vi "Write Current Waveform to Log Instances.vi"(6 "Current Wfm":T1, 8 "error in (no error)":errorcluster, 9 "Data in":dbl[](array[numeric]), 10 "Wfm Index":i32, 11 "Waveform Log in":refnum<class "Waveform Log.lvclass">) -> (0 "error out":errorcluster, 1 "Data out":dbl[](array[numeric]), 3 "Waveform Log out":refnum<class "Waveform Log.lvclass">)   [LabVIEW 2015, in "Waveform Data Logger Engine.lvlib" / "Waveform Log.lvclass"]
uses:
  Waveform Log.lvclass
  Waveform Receive/Wfm Info.ctl
  Waveform Log.lvclass/Waveform Log.ctl
  Logs/Segmented Logs/Segmented Log/Segmented Log.lvclass/Segmented Log.ctl
  Shared/Classes/Log File Specifications/Log File Specification/Log File Specification.lvclass/Log File Specification.ctl
  Shared/Classes/Log File Specifications/Waveform TDMS Log File Specification/Waveform TDMS Log File Specification.lvclass/Waveform TDMS Log File Specification.ctl
  Logs/Log Files/Log File/Log File.lvclass/Log File.ctl
  Logs/Log Files/TDMS Log File/TDMS Log File.lvclass/TDMS Log File.ctl
  Logs/Log Files/Text Log File/Text Log File.lvclass/Text Log File.ctl
  Logs/Segmented Logs/Footprint Segmented Log/Footprint Segmented Log.lvclass/Footprint Segmented Log.ctl
  Logs/Segmented Logs/Time Segmented Log/Time Segmented Log.lvclass/Time Segmented Log.ctl
  Logs/Segmented Logs/Segmented Log/Write Waveform to Log File Instance.vi
  Shared/Classes/Log File Specifications/Log File Specification/Get Log Specification Type.vi
  Shared/Classes/Log File Specifications/Waveform TDMS Log File Specification/Get Current Group.vi
  Logs/Log Files/Log File/Get Log File Type.vi
  Logs/Log Files/Log File/Write Channel to Log File.vi
  Logs/Log Files/TDMS Log File/Set TDMS Channel Property.vi
  Logs/Log Files/TDMS Log File/Copy Channel Properties.vi
  Logs/Segmented Logs/Segmented Log/Check Close File.vi
  Logs/Segmented Logs/Segmented Log/Check Open File.vi
  Logs/Log Files/TDMS Log File/Write Channel to TDMS Log File.vi
  Logs/Log Files/Text Log File/Write Channel to Text Log File.vi
  Logs/Segmented Logs/Segmented Log/Close Log File Instance.vi
  Logs/Segmented Logs/Segmented Log/Segment Log File.vi
  Logs/Segmented Logs/Segmented Log/Open Log File Instance.vi
  Logs/Log Files/Log File/Close Log File.vi
  Logs/Segmented Logs/Segmented Log/Make File Read-Only.vi
  Logs/Segmented Logs/Segmented Log/On Segmented Log Complete.vi
  Logs/Segmented Logs/Segmented Log/On File Close.vi
  Logs/Segmented Logs/Footprint Segmented Log/Segment Log File (Footprint).vi
  Logs/Segmented Logs/Time Segmented Log/Segment Log File (Time).vi
  Shared/Classes/Log File Specifications/Log File Specification/Open Log File.vi
  Shared/Classes/Log File Specifications/Log File Specification/Set Path Tag.vi
  Logs/Segmented Logs/Segmented Log/On File Open.vi
  Shared/Classes/Log File Specifications/Log File Specification/Set Filename Offset.vi
  Logs/Log Files/TDMS Log File/Close TDMS Log File.vi
  Logs/Log Files/Text Log File/Close Text Log File.vi
  Logs/Segmented Logs/Segmented Log/Get Current Log File Instance.vi
  Logs/Log Files/Log File/Get File Size.vi
  Logs/Log Files/Log File/Get Start Time.vi
  Shared/Classes/Log File Specifications/Log File Specification/Build File Path.vi
  Shared/Classes/Log File Specifications/Log File Specification/Resolve File Conflicts.vi
  <vilib>/Utility/error.llb/Error Cluster From Error Code.vi
  Shared/Classes/Log File Specifications/Log File Specification/Initialize Log File.vi
  <vilib>/Utility/libraryn.llb/Create Directory Recursive.vi
  <vilib>/Utility/libraryn.llb/Check if File or Folder Exists.vi
  <vilib>/Utility/libraryn.llb/Get File Extension.vi
  Logs/Log Files/Text Log File/Text Log File.lvclass
  Logs/Log Files/TDMS Log File/TDMS Log File.lvclass
  Logs/Log Files/Log File/Log File.lvclass
  Logs/Segmented Logs/Time Segmented Log/Time Segmented Log.lvclass
  Logs/Segmented Logs/Footprint Segmented Log/Footprint Segmented Log.lvclass
  Shared/Classes/Log File Specifications/Waveform TDMS Log File Specification/Waveform TDMS Log File Specification.lvclass
  Waveform Receive/Waveform Receive.lvclass
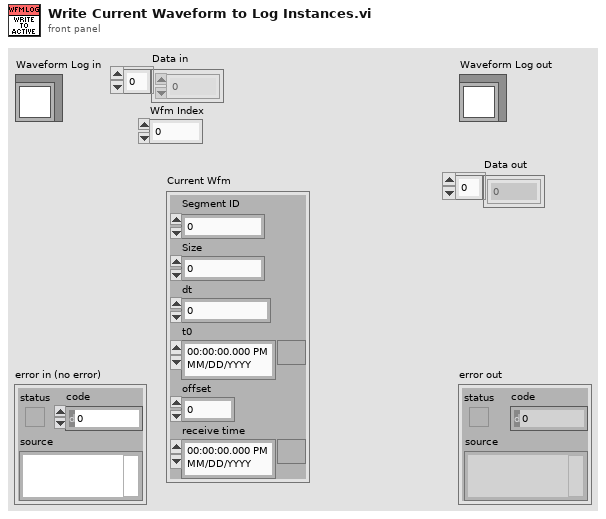
[diagram p1: front panel]
types:
  T1 = typedef "Waveform Data Logger Engine.lvlib/Waveform Receive.lvclass/Wfm Info.ctl" = cluster{"Segment ID":u64, "Size":i32, "dt":dbl, "t0":timestamp, "offset":u64, "receive time":timestamp}
  T2 = typedef "Waveform Data Logger Engine.lvlib/Waveform Log.lvclass/Log Instance.ctl" = cluster{"Segmented Log":refnum<data-value>, "Log Waveforms":T3[], "Log Start":timestamp, "Log Stop":timestamp, "Start Trigger Time":timestamp, "Stop Trigger Time":timestamp, "Time of Last Write":timestamp, "Timeout":dbl, "Stop cmd received":bool}
  T3 = typedef "Waveform Data Logger Engine.lvlib/Waveform Log.lvclass/Log Instance Waveform.ctl" = cluster{"Wfm Info":T4, "Count / Instance":i32, "Previous Segment":u64, "Wfm Complete?":bool, "Last Sample Logged":timestamp, "Data Logged":bool, "Log segmented":bool}
  T4 = typedef "Waveform Data Logger Engine.lvlib/Waveform Log.lvclass/Waveform Information.ctl" = cluster{"Name":string, "Wfm Data Type":T5, "Decimation":u32}
  T5 = typedef "Waveform Data Logger Engine.lvlib/Waveform Log.lvclass/Waveform Data Type.ctl" = enum16{"Double", "ComplexDouble"}
  T6 = typedef "Waveform Data Logger Engine.lvlib/Waveform Log.lvclass/Waveform Log Wfm Meta Data.ctl" = cluster{"Segment ID":u64, "dt":dbl, "t0":timestamp, "tf":timestamp}
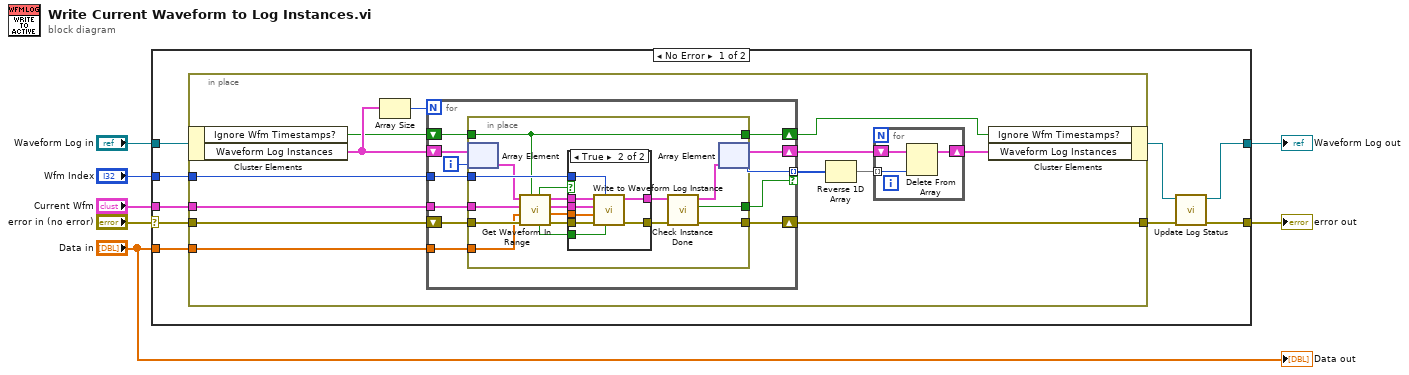
[diagram p0: block diagram]
diagram:
  n1 = case shown="No Error" "error in (no error)" {
    selector: "error in (no error)" -> [w15 w73]
    tunnel: [w8 w73] -> w6
    tunnel: [w9 w72] -> w4
    tunnel: "Waveform Log in" -> [w12 w72]
    tunnel: "Wfm Index" -> [w16 _]
    tunnel: "Data in" -> [w14 _]
    tunnel: "Current Wfm" -> [w13 _]
    frame No Error {
      n2 = in-place {
        in-place-border: w16 -> [w29]
        in-place-border: w15 -> [w28]
        in-place-border: [w17] -> w10
        in-place-border: w14 -> [w27]
        in-place-border: w13 -> [w25]
        n3 = in-place-cluster #1(w12) -> ("Ignore Wfm Timestamps?"=w23:bool, "Waveform Log Instances"=w24:T2[])
        n4 = Array Size(array=w24) -> (size(s)=w26:i32)
        n5 = for {
          N: w26 -> [_]
          tunnel: w29 -> [w44]
          tunnel: w27 -> [w39]
          shift-right: [w36] -> w17
          shift-left: w28 -> [w43]
          tunnel: w25 -> [w42]
          shift-right: [w35] -> w19
          shift-left: w24 -> [w41]
          shift-right: [w37] -> w22
          shift-left: w23 -> [w38]
          tunnel: [w34] -> w20 mode=indexing if=w33
          i -> [w40]
          n6 = in-place {
            in-place-border: w44 -> [w61]
            in-place-border: w43 -> [w60]
            in-place-border: w42 -> [w56]
            in-place-border: w39 -> [w53]
            in-place-border: w38 -> [w52]
            in-place-border: [w52] -> w37
            in-place-border: [w48] -> w36
            in-place-border: [w47] -> w33
            n7 = in-place-array #2(w41, w40) -> (w55:T2)
            n8 = call "Get Waveform In Range.vi"("Ignore Wfm Timestamps?"=w52, "error in (no error)"=w60, "Data in"=w53, "Waveform Info"=w56, "Log Instance in"=w55) -> ("error out"=w59:errorcluster, "Data out"=w58:dbl[], "Waveform Data"=w57:T6, "Log Instance out"=w54:T2, "tf Modified?"=w45:bool, "In Range?"=w46:bool)  [unwired: 1 in]
            n9 = case shown="True" w46 {
              tunnel: w61 -> [_ w66]
              tunnel: [w63 w71] -> w50
              tunnel: w59 -> [w63 w70]
              tunnel: w58 -> [_ w67]
              tunnel: w57 -> [_ w68]
              tunnel: w54 -> [w62 w69]
              tunnel: [w62 w65] -> w51
              tunnel: w45 -> [_ w64]
              frame False {
              }
              frame True {
                n10 = call "Write to Waveform Log Instance.vi"("tf Modified?"=w64, "Wfm Index"=w66, "error in (no error)"=w70, "Data"=w67, "Waveform Data"=w68, "Log Instance in"=w69) -> ("error out"=w71:errorcluster, "Log Instance out"=w65:T2)  [unwired: 4 in]
              }
            }
            n11 = call "Check Instance Done.vi"("error in (no error)"=w50, "Log Instance in"=w51) -> ("error out"=w48:errorcluster, "Done?"=w47:bool, "Log Instance out"=w49:T2)  [unwired: 7 in]
            n12 = in-place-array #2(w49) -> (w35:T2[], w34:i32)
          }
        }
        n13 = Reverse 1D Array(array=w20) -> (reversed array=w21:i32[])
        n14 = for {
          shift-right: [w31] -> w18
          shift-left: w19 -> [w32]
          tunnel: w21 -> [w30] mode=indexing
          n15 = Delete From Array(array=w32, index=w30) -> (array with subset deleted=w31:T2[])  [unwired: 1 in, 1 out]
        }
        n16 = in-place-cluster #1("Ignore Wfm Timestamps?"=w22, "Waveform Log Instances"=w18) -> (w11:refnum<class "Waveform Log.lvclass">)
      }
      n17 = call "Update Log Status.vi"("error in (no error)"=w10, "Waveform Log in"=w11) -> ("error out"=w8:errorcluster, "Waveform Log out"=w9:refnum<class "Waveform Log.lvclass">)  [unwired: 8 in]
    }
    frame Error {
    }
  }
  "error out" <- w6
  "Waveform Log out" <- w4
  "Data out" <- "Data in"
